vi "Kontaktpositionen_finden.vi"(8 "Fehler in":errorcluster, 10 "Größe Kontaktsuchfeld":sgl=50.0, 11 "Cluster in":T1={"Initialisierung"={"Online?"=FALSE, "Grundpfad"=path "", "Kamera Oben"="", "IP-Adresse Flüssiglinse"="", "Flüssiglinse"=refnum, "Kamera Unten"="", "IP-Adresse SPS"="", "SPS-Verbindung"={"TCP Connection Ref"=refnum, "IP address"="", "timeout ms"=5000, "Connected?"=FALSE, "PLC Type"=enum."S7 1200", "Rack S7 400"=0, "Slot S7 400"=0, "PDU Size"=0, "connection semaphore"=refnum}, "IP-Adresse Lichtgitter"="", "Lichtgitter"=refnum, "Skalierungsfaktor"=0.0, "Bilder Oben"=[], "Bild Unten"=refnum, "Bild Ausschnitt Unten"=refnum}, "Einstellungen"={"Gesamtablauf gestartet"=FALSE, "i. O. Bilder speichern"=FALSE, "Bildspeicherung Offline"=FALSE, "Ausgewähltes Offline-Datum"="", "Ausgewähltes Offline-Teil"="", "Speicherpfad Bilder"=path ""}, "Artikeldaten"={"Artikelnummer"="", "Fertigungsauftrag"="", "Muster ISO"=refnum, "Belichtungszeit Referenzmarken"=0.0, "Fokus Referenzmarken"=0.0, "Belichtungszeit ISO"=0.0, "Fokus ISO"=0.0, "Belichtungszeit Unten"=0.0, "Kontaktanzahl"=0, "Aktueller Kontakt"=0, "Kontaktposition"={"x"=0.0, "y"=0.0}, "Winkel ISO"=0.0, "ISO-Muster nicht vorhanden"=FALSE}, "Werte Kamera Oben"={"Koordinatensystem"={"Punkt x-Achse"={"X"=0.0, "Y"=0.0}, "Ursprung"={"X"=0.0, "Y"=0.0}, "Punkt y-Achse"={"X"=0.0, "Y"=0.0}}, "Position Kontakt"={"x"=0.0, "y"=0.0}, "Winkel Kontakt"=0.0}, "Werte Kamera Unten"={"Prüfung Unten n. i. O."=FALSE}, "Werte Lichtgitter"={"Messwerte Referenzmarken"=[], "Mittelpunkt Referenzmarken"={"x"=0.0, "y"=0.0}, "Messwerte Kontakt"=[], "Offset"={"x"=0.0, "y"=0.0}}, "Rückmeldungen"={"Koordinaten ermittelt"=FALSE, "Vermessung Lichtgitter fertig"=FALSE, "Nachkontrolle Kamera Unten fertig"=FALSE}, "Fehler"={"Referenzen nicht gefunden"=FALSE, "Kontakt nicht gefunden"=FALSE, "Referenzen nicht in Lichtgitter"=FALSE, "Kontakt zu groß"=FALSE, "Kontakt zu klein"=FALSE}, "Statistik"={"Statistiken"=[]}, "Timer"={"Timer Start Position"=0, "Timer Start Lichtgitter"=0, "Timer Start Kamera Unten"=0}}) -> (0 "Fehler out":errorcluster, 1 "Durchmesser Loch":dbl, 2 "Kontakt nicht gefunden":bool, 3 "Cluster out":T1={"Initialisierung"={"Online?"=FALSE, "Grundpfad"=path "", "Kamera Oben"="", "IP-Adresse Flüssiglinse"="", "Flüssiglinse"=refnum, "Kamera Unten"="", "IP-Adresse SPS"="", "SPS-Verbindung"={"TCP Connection Ref"=refnum, "IP address"="", "timeout ms"=5000, "Connected?"=FALSE, "PLC Type"=enum."S7 1200", "Rack S7 400"=0, "Slot S7 400"=0, "PDU Size"=0, "connection semaphore"=refnum}, "IP-Adresse Lichtgitter"="", "Lichtgitter"=refnum, "Skalierungsfaktor"=0.0, "Bilder Oben"=[], "Bild Unten"=refnum, "Bild Ausschnitt Unten"=refnum}, "Einstellungen"={"Gesamtablauf gestartet"=FALSE, "i. O. Bilder speichern"=FALSE, "Bildspeicherung Offline"=FALSE, "Ausgewähltes Offline-Datum"="", "Ausgewähltes Offline-Teil"="", "Speicherpfad Bilder"=path ""}, "Artikeldaten"={"Artikelnummer"="", "Fertigungsauftrag"="", "Muster ISO"=refnum, "Belichtungszeit Referenzmarken"=0.0, "Fokus Referenzmarken"=0.0, "Belichtungszeit ISO"=0.0, "Fokus ISO"=0.0, "Belichtungszeit Unten"=0.0, "Kontaktanzahl"=0, "Aktueller Kontakt"=0, "Kontaktposition"={"x"=0.0, "y"=0.0}, "Winkel ISO"=0.0, "ISO-Muster nicht vorhanden"=FALSE}, "Werte Kamera Oben"={"Koordinatensystem"={"Punkt x-Achse"={"X"=0.0, "Y"=0.0}, "Ursprung"={"X"=0.0, "Y"=0.0}, "Punkt y-Achse"={"X"=0.0, "Y"=0.0}}, "Position Kontakt"={"x"=0.0, "y"=0.0}, "Winkel Kontakt"=0.0}, "Werte Kamera Unten"={"Prüfung Unten n. i. O."=FALSE}, "Werte Lichtgitter"={"Messwerte Referenzmarken"=[], "Mittelpunkt Referenzmarken"={"x"=0.0, "y"=0.0}, "Messwerte Kontakt"=[], "Offset"={"x"=0.0, "y"=0.0}}, "Rückmeldungen"={"Koordinaten ermittelt"=FALSE, "Vermessung Lichtgitter fertig"=FALSE, "Nachkontrolle Kamera Unten fertig"=FALSE}, "Fehler"={"Referenzen nicht gefunden"=FALSE, "Kontakt nicht gefunden"=FALSE, "Referenzen nicht in Lichtgitter"=FALSE, "Kontakt zu groß"=FALSE, "Kontakt zu klein"=FALSE}, "Statistik"={"Statistiken"=[]}, "Timer"={"Timer Start Position"=0, "Timer Start Lichtgitter"=0, "Timer Start Kamera Unten"=0}})   [LabVIEW 2024]
uses:
  Cluster.ctl
  Kontaktmontagemodul.exe/1abvi3w/vi.lib/userDefined/High Color/IMAQdx.ctl
  Kontaktmontagemodul.exe/1abvi3w/vi.lib/DATA AHEAD/SP7/typedefs/S7 Connection.ctl
  Kontaktmontagemodul.exe/1abvi3w/vi.lib/DATA AHEAD/SP7/typedefs/PLC Type.ctl
  Kontaktmontagemodul.exe/1abvi3w/vi.lib/vision/Image Controls.llb/IMAQ Image.ctl
  Koordinatensystem.ctl
  Statistik.ctl
  Kontaktmontagemodul.exe/1abvi3w/vi.lib/vision/Pattern Matching.llb/IMAQ Curve Parameters.ctl
  Kontaktmontagemodul.exe/1abvi3w/vi.lib/vision/NI_Vision_Development_Module.lvlib
  Kontaktmontagemodul.exe/1abvi3w/vi.lib/DATA AHEAD/SP7/SP7.lvlib
panel:
  in  "Winkel korrigieren?":bool=TRUE
  out "Winkelversatz soll/ist":dbl format="%#.3f"
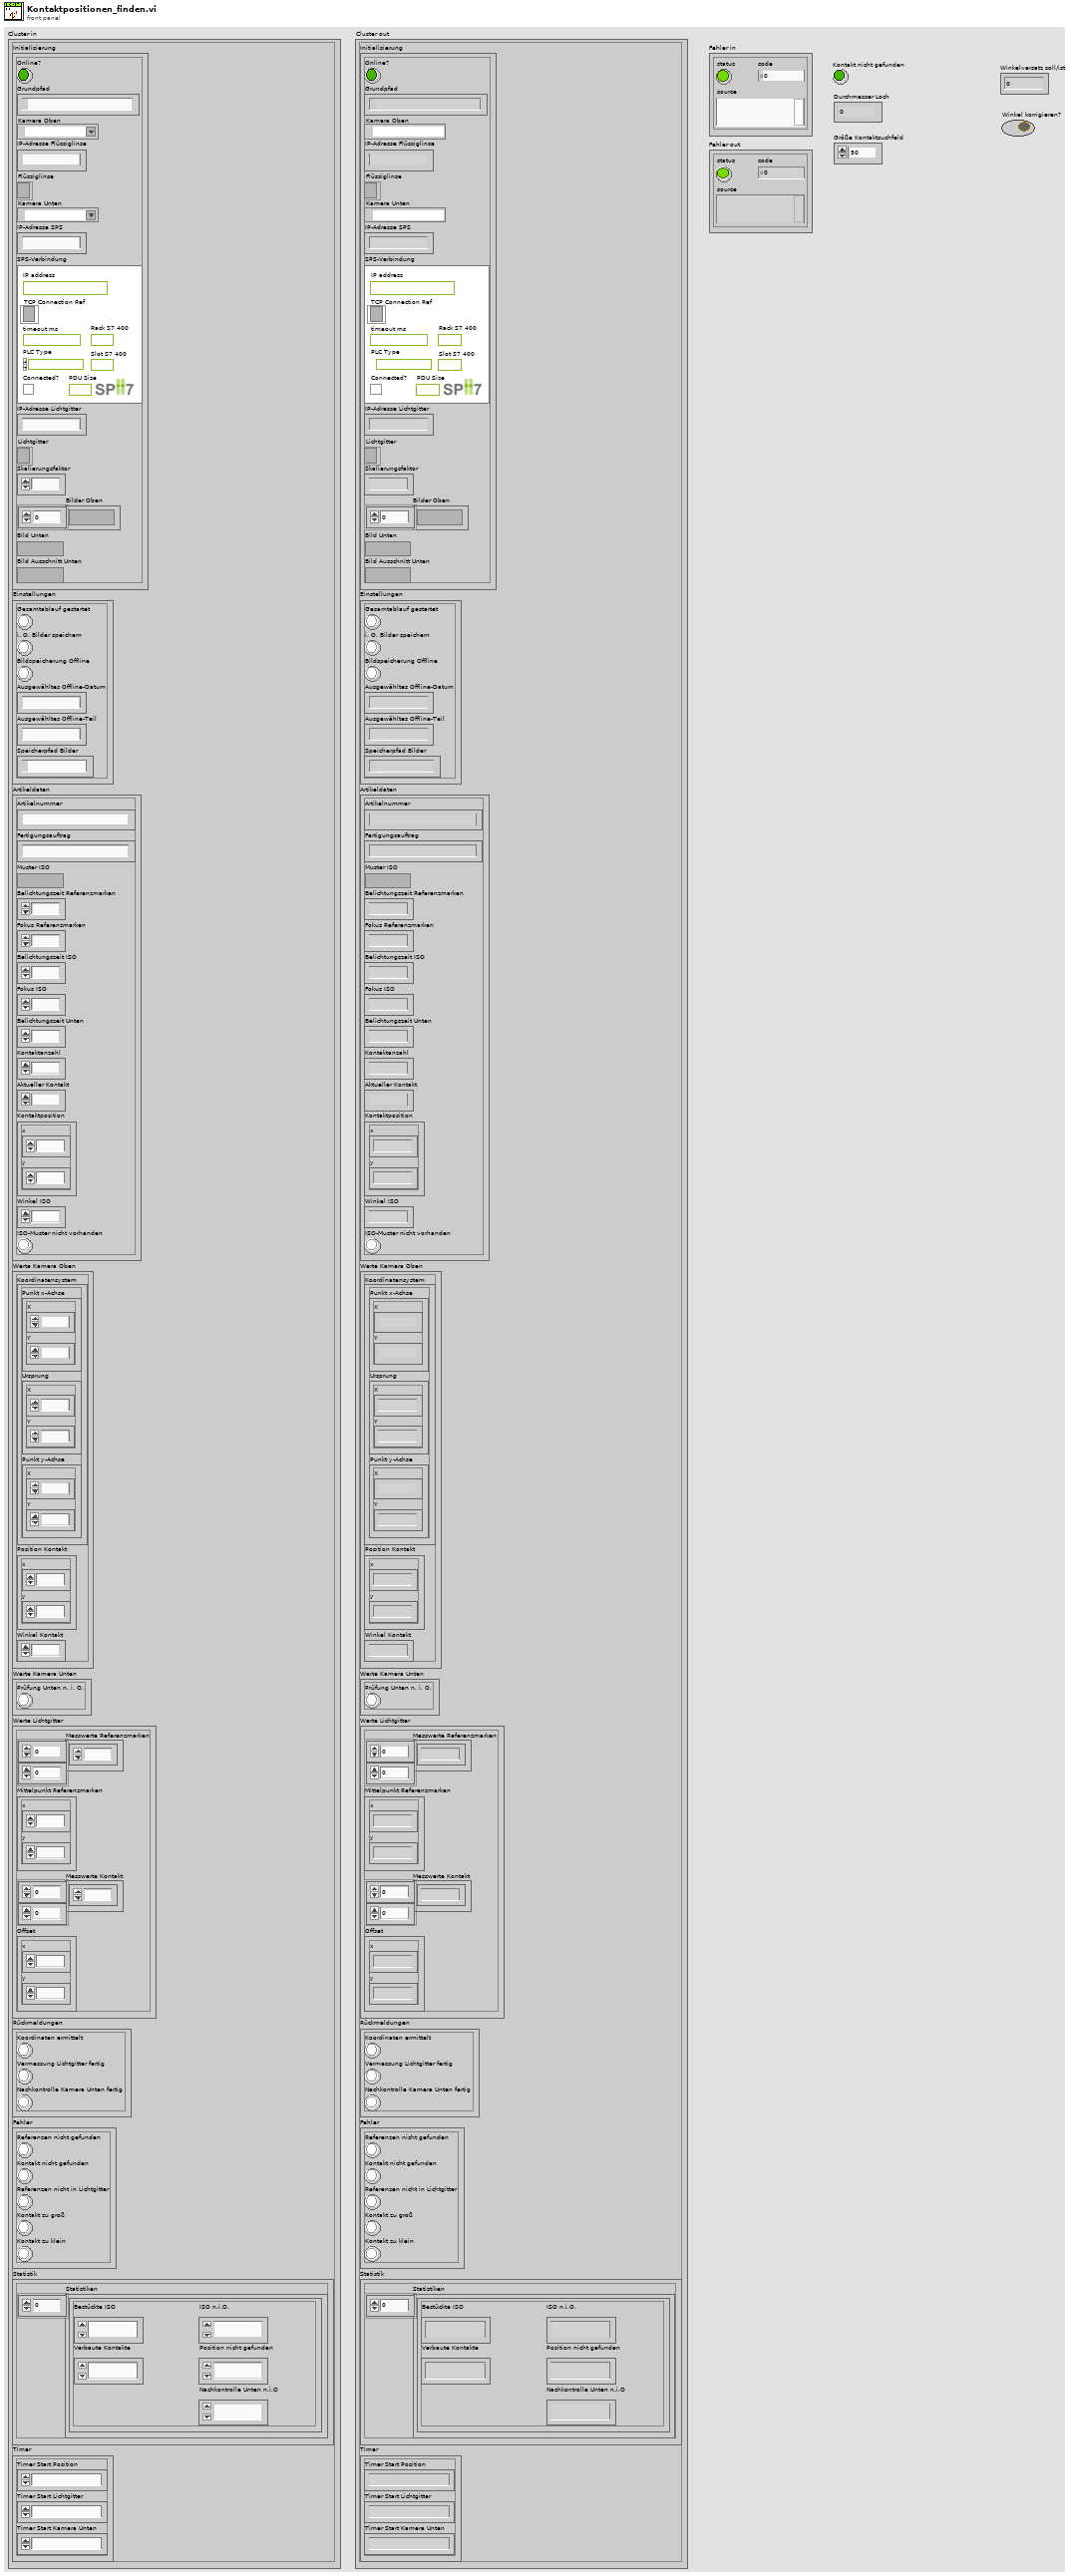
[diagram p1: front panel]
types:
  T1 = typedef "Cluster.ctl" = cluster{"Initialisierung":cluster{"Online?":bool, "Grundpfad":path, "Kamera Oben":T2, "IP-Adresse Flüssiglinse":string, "Flüssiglinse":refnum<k5>, "Kamera Unten":T2, "IP-Adresse SPS":string, "SPS-Verbindung":T3, "IP-Adresse Lichtgitter":string, "Lichtgitter":refnum<k5>, "Skalierungsfaktor":dbl, "Bilder Oben":T6[], "Bild Unten":T6, "Bild Ausschnitt Unten":T6}, "Einstellungen":cluster{"Gesamtablauf gestartet":bool, "i. O. Bilder speichern":bool, "Bildspeicherung Offline":bool, "Ausgewähltes Offline-Datum":string, "Ausgewähltes Offline-Teil":string, "Speicherpfad Bilder":path}, "Artikeldaten":cluster{"Artikelnummer":string, "Fertigungsauftrag":string, "Muster ISO":T6, "Belichtungszeit Referenzmarken":dbl, "Fokus Referenzmarken":dbl, "Belichtungszeit ISO":dbl, "Fokus ISO":dbl, "Belichtungszeit Unten":dbl, "Kontaktanzahl":u32, "Aktueller Kontakt":i16, "Kontaktposition":cluster{"x":sgl, "y":sgl}, "Winkel ISO":sgl, "ISO-Muster nicht vorhanden":bool}, "Werte Kamera Oben":cluster{"Koordinatensystem":T7, "Position Kontakt":cluster{"x":dbl, "y":dbl}, "Winkel Kontakt":dbl}, "Werte Kamera Unten":cluster{"Prüfung Unten n. i. O.":bool}, "Werte Lichtgitter":cluster{"Messwerte Referenzmarken":dbl[][], "Mittelpunkt Referenzmarken":cluster{"x":dbl, "y":dbl}, "Messwerte Kontakt":dbl[][], "Offset":cluster{"x":dbl, "y":dbl}}, "Rückmeldungen":cluster{"Koordinaten ermittelt":bool, "Vermessung Lichtgitter fertig":bool, "Nachkontrolle Kamera Unten fertig":bool}, "Fehler":cluster{"Referenzen nicht gefunden":bool, "Kontakt nicht gefunden":bool, "Referenzen nicht in Lichtgitter":bool, "Kontakt zu groß":bool, "Kontakt zu klein":bool}, "Statistik":cluster{"Statistiken":T8[]}, "Timer":cluster{"Timer Start Position":u32, "Timer Start Lichtgitter":u32, "Timer Start Kamera Unten":u32}}
  T2 = typedef "IMAQdx.ctl" = refnum<k21>
  T3 = typedef "SP7.lvlib/S7 Connection.ctl" = cluster{"TCP Connection Ref":refnum<k5>, "IP address":string, "timeout ms":i32, "Connected?":bool, "PLC Type":T4, "Rack S7 400":u8, "Slot S7 400":u8, "PDU Size":u16, "connection semaphore":T5}
  T4 = typedef "SP7.lvlib/PLC Type.ctl" = enum16{"S7 200", "S7 300/400", "S7 1200", "S7 1500", "LOGO!8"}
  T5 = typedef "Semaphore RefNum" = refnum<k1>
  T6 = typedef "IMAQ Image.ctl" = refnum<image>
  T7 = typedef "Koordinatensystem.ctl" = cluster{"Punkt x-Achse":cluster{"X":sgl, "Y":sgl}, "Ursprung":cluster{"X":sgl, "Y":sgl}, "Punkt y-Achse":cluster{"X":sgl, "Y":sgl}}
  T8 = typedef "Statistik.ctl" = cluster{"Bestückte ISO":u32, "Verbaute Kontakte":u32, "ISO n.i.O.":u32, "Nachkontrolle Unten n.i.O":u32, "Position nicht gefunden":u32}
  T9 = typedef "IMAQ Curve Parameters.ctl" = cluster{"Extraction Mode":u32, "Edge Threshold":i32, "Edge Filter Size":u32, "Min Length":i32, "Row Search Step Size":i32, "Col Search Step Size":i32, "Max Endpoint Gap":i32, "Closed":bool, "Subpixel":bool}
  T10 = typedef "IMAQ Rectangle" = cluster{"Left":i32, "Top":i32, "Right":i32, "Bottom":i32, "Rotation":dbl}
  T11 = typedef "ROI Descriptor" = cluster{"Global Rectangle":i32[], "Contours":cluster{"ID":enum32{"External", "Internal"}, "Type":u32, "Coordinates":i32[]}[]}
  T12 = cluster{"Position":cluster{"X":sgl, "Y":sgl}, "Radius":dbl, "Score":dbl}[]
  T13 = cluster{"Farbe Kreis":u32, "Kreis ausfüllen?":bool, "Bounding Rechteck anzeigen?":bool, "Farbe Bounding Rechteck":u32}
  T14 = cluster{"Position":cluster{"X":sgl, "Y":sgl}, "Radius":dbl, "Score":dbl}
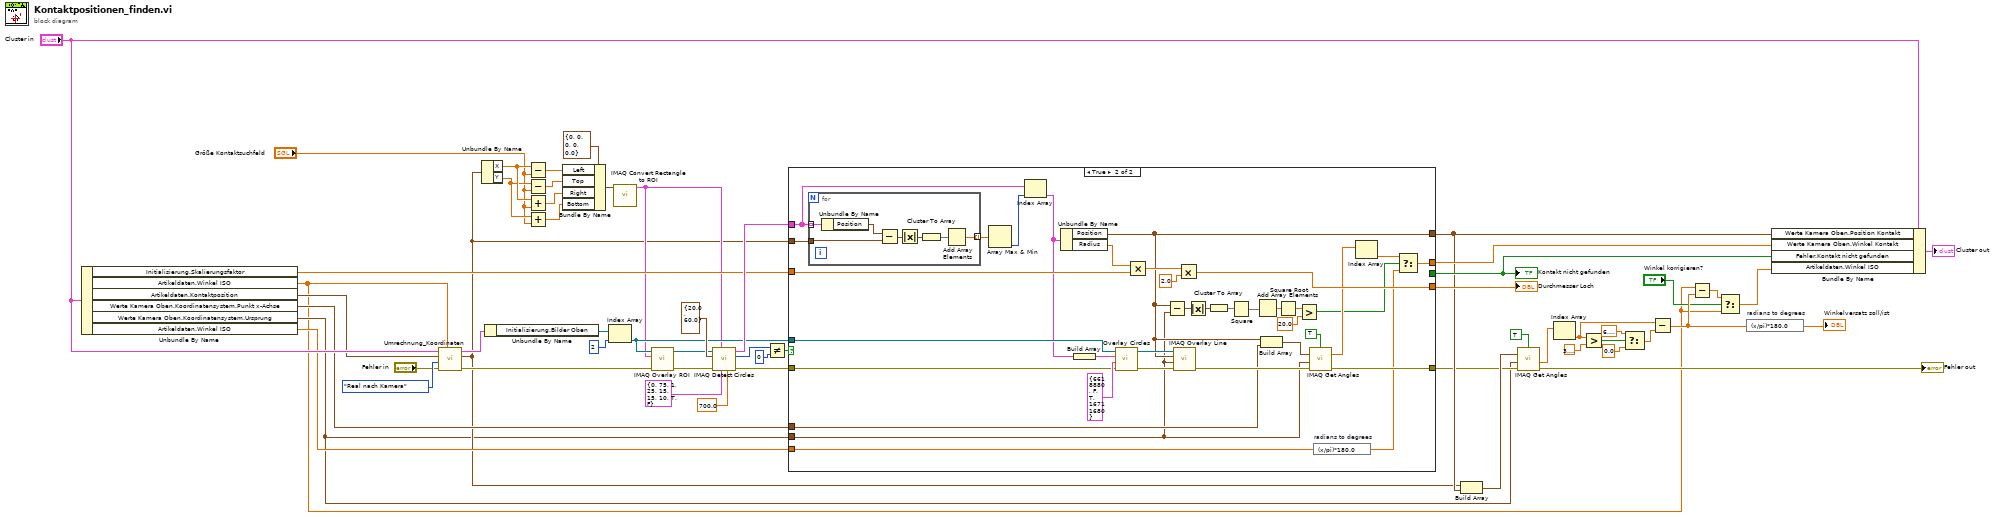
[diagram p0: block diagram]
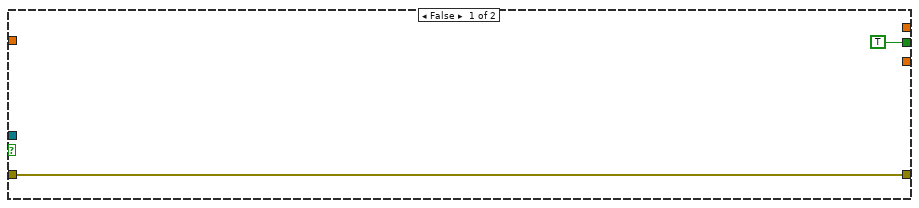
[diagram p2: hidden frame]
diagram:
  n1 = Unbundle By Name("Cluster in") -> ("Initialisierung.Skalierungsfaktor"=w30:dbl, "Artikeldaten.Winkel ISO"=w1:sgl, "Artikeldaten.Kontaktposition"=w19:cluster{"x":sgl, "y":sgl}, "Werte Kamera Oben.Koordinatensystem.Punkt x-Achse"=w29:cluster{"X":sgl, "Y":sgl}, "Werte Kamera Oben.Koordinatensystem.Ursprung"=w3:cluster{"X":sgl, "Y":sgl}, "Artikeldaten.Winkel ISO"=w27:sgl)
  n2 = call "Umrechnung_Koordinaten.vi"("Anderer Winkel"=w1, "error in"="Fehler in", "Richtung"=enum16{"Kamera nach Real", "Real nach Kamera"}."Real nach Kamera", "Koordinaten in"=w19, "Cluster in"="Cluster in") -> ("error out"=w39:errorcluster, "Koordinaten out"=w17:cluster{"X":sgl, "Y":sgl}, "Cluster out"=w51:T1)  [unwired: 4 in]
  n3 = Unbundle By Name(w17) -> ("X"=w45:sgl, "Y"=w44:sgl)
  n4 = Unbundle By Name(w51) -> ("Initialisierung.Bilder Oben"=w54:T6[])
  n5 = Subtract(x=w45, y="Größe Kontaktsuchfeld") -> (x-y=w46:sgl)
  n6 = Subtract(x=w44, y="Größe Kontaktsuchfeld") -> (x-y=w43:sgl)
  n7 = Add(x=w45, y="Größe Kontaktsuchfeld") -> (x+y=w42:sgl)
  n8 = Add(x=w44, y="Größe Kontaktsuchfeld") -> (x+y=w41:sgl)
  n9 = Bundle By Name(cluster=T10 {"Left"=0, "Top"=0, "Right"=0, "Bottom"=0, "Rotation"=0.0} ("Rectangle"), "Left"=w46, "Top"=w43, "Right"=w42, "Bottom"=w41) -> (w47:T10)
  n10 = Index Array(array=w54, index=2 ("t")) -> (element=w26:T6)
  n11 = call "IMAQ Convert Rectangle to ROI"("Rectangle"=w47) -> ("ROI Descriptor"=w25:T11)  [unwired: 8 in, 1 out]
  n12 = call "IMAQ Overlay ROI"("error in (no error)"=w39, "ROI Descriptor"=w25, "Image"=w26) -> ("error out"=w38:errorcluster, "Image Out"=w37:T6)  [unwired: 7 in]
  n13 = call "IMAQ Detect Circles"("Minimum match score"=700.0, "Curve Parameters"=T9 {"Extraction Mode"=0, "Edge Threshold"=75, "Edge Filter Size"=1, "Min Length"=25, "Row Search Step Size"=15, "Col Search Step Size"=15, "Max Endpoint Gap"=10, "Closed"=TRUE, "Subpixel"=FALSE}, "ROI Descriptor"=w25, "error in (no error)"=w38, "Circle Descriptor"=cluster{"Min Radius":dbl, "Max Radius":dbl} {"Min Radius"=20.0, "Max Radius"=60.0}, "Image"=w37) -> ("error out"=w36:errorcluster, "Number of Matches Returned"=w23:i32, "Circles"=w35:T12)  [unwired: 3 in]
  n14 = Not Equal?(x=w23, y=0) -> (x != y?=w33:bool)
  n15 = case shown="True" w33 {
    tunnel: [w58 w81] -> w5
    tunnel: [_ w76] -> w20
    tunnel: w3 -> [_ w75]
    tunnel: w30 -> [_ w89]
    tunnel: [_ w86] -> w40
    tunnel: w26 -> [_ w85]
    tunnel: w36 -> [w58 w84]
    tunnel: w35 -> [_ w60]
    tunnel: [TRUE ("Kontakt nicht gefunden") _] -> w22
    tunnel: w29 -> [_ w79]
    tunnel: [_ w66] -> w28
    tunnel: w27 -> [_ w65]
    tunnel: w17 -> [_ w62]
    frame False {
    }
    frame True {
      n16 = for {
        tunnel: w60 -> [w101] mode=indexing
        tunnel: w62 -> [w98]
        tunnel: [w95] -> w61 mode=indexing
        n17 = Unbundle By Name(w101) -> ("Position"=w99:cluster{"X":sgl, "Y":sgl})
        n18 = Subtract(x=w99, y=w98) -> (x-y=w100:cluster{"X":sgl, "Y":sgl})
        n19 = Absolute Value(x=w100) -> (abs(x)=w97:cluster{"X":sgl, "Y":sgl})
        n20 = Cluster To Array(cluster=w97) -> (array=w96:sgl[])
        n21 = Add Array Elements(numeric array=w96) -> (sum=w95:sgl)
      }
      n22 = Array Max & Min(array=w61) -> (min index (indices)=w59:i32)  [unwired: 3 out]
      n23 = Index Array(array=w60, index=w59) -> (element=w63:T14)
      n24 = Unbundle By Name(w63) -> ("Position"=w76:cluster{"X":sgl, "Y":sgl}, "Radius"=w90:dbl)
      n25 = Build Array(w63) -> (w94:T12)
      n26 = call "Overlay Circles.vi"("error in"=w84, "Einstellungen"=T13 {"Farbe Kreis"=6618880, "Kreis ausfüllen?"=FALSE, "Bounding Rechteck anzeigen?"=TRUE, "Farbe Bounding Rechteck"=16711680}, "Circles"=w94, "Image in"=w85) -> ("error out"=w92:errorcluster, "Image out"=w91:T6)  [unwired: 6 in]
      n27 = Multiply(x=w90, y=w89) -> (x*y=w88:dbl)
      n28 = Subtract(x=w76, y=w75) -> (x-y=w77:cluster{"X":sgl, "Y":sgl})
      n29 = call "IMAQ Overlay Line"("error in (no error)"=w92, "End Point"=w75, "Start Point"=w76, "Image"=w91) -> ("error out"=w82:errorcluster)  [unwired: 6 in, 1 out]
      n30 = Multiply(x=w88, y=2.0) -> (x*y=w86:dbl)
      n31 = Absolute Value(x=w77) -> (abs(x)=w74:cluster{"X":sgl, "Y":sgl})
      n32 = Cluster To Array(cluster=w74) -> (array=w72:sgl[])
      n33 = Square(x=w72) -> (x^2=w73:sgl[])
      n34 = Add Array Elements(numeric array=w73) -> (sum=w71:sgl)
      n35 = Build Array(w76, w79) -> (w80:cluster{"X":sgl, "Y":sgl}[])
      n36 = Square Root(x=w71) -> (sqrt(x)=w70:sgl)
      n37 = Greater?(x=w70, y=sgl 20.0) -> (0:w68:bool)
      n38 = call "IMAQ Get Angles"("error in (no error)"=w82, "Vertex"=w75, "Points"=w80, "Use Vertex (No)"=TRUE) -> ("error out"=w81:errorcluster, "Angles (deg)"=w78:sgl[])  [unwired: 1 in, 1 out]
      n39 = expression code="(x/pi)*180.0" "radians to degrees"(w65) -> (w64:sgl)
      n40 = Index Array(array=w78) -> (element=w67:sgl)  [unwired: 1 in]
      n41 = Select(t=w67, s=w68, f=w64) -> (s? t:f=w66:sgl)
    }
  }
  "Kontakt nicht gefunden" <- w22
  "Durchmesser Loch" <- w40
  n42 = Build Array(w17, w20) -> (w18:cluster{"X":sgl, "Y":sgl}[])
  n43 = call "IMAQ Get Angles"("error in (no error)"=w5, "Vertex"=w3, "Points"=w18, "Use Vertex (No)"=TRUE) -> ("error out"=→"Fehler out":errorcluster, "Angles (rad)"=w16:sgl[])  [unwired: 1 in, 1 out]
  n44 = Index Array(array=w16) -> (element=w11:sgl)  [unwired: 1 in]
  n45 = Greater?(x=w11, y=3.141592653589793) -> (0:w14:bool)
  n46 = Select(t=6.283185307179586, s=w14, f=0.0) -> (s? t:f=w10:dbl)
  n47 = Subtract(x=w11, y=w10) -> (x-y=w8:dbl)
  n48 = Subtract(x=w1, y=w8) -> (x-y=w6:dbl)
  n49 = Select(t=w6, s="Winkel korrigieren?", f=w1) -> (s? t:f=w2:dbl)
  n50 = expression code="(x/pi)*180.0" "radians to degrees"(w8) -> (→"Winkelversatz soll/ist":dbl)
  n51 = Bundle By Name(cluster="Cluster in", "Werte Kamera Oben.Position Kontakt"=w20, "Werte Kamera Oben.Winkel Kontakt"=w28, "Fehler.Kontakt nicht gefunden"=w22, "Artikeldaten.Winkel ISO"=w2) -> (→"Cluster out":T1)
